vi "sub_result-log.vi"(7 "data":enum16{"header", "result"}(ring), 11 "text":string) -> ()   [LabVIEW 2019]
uses:
  _ctrl/rw.ctl
panel:
  out "path":path
  out "error out":errorcluster
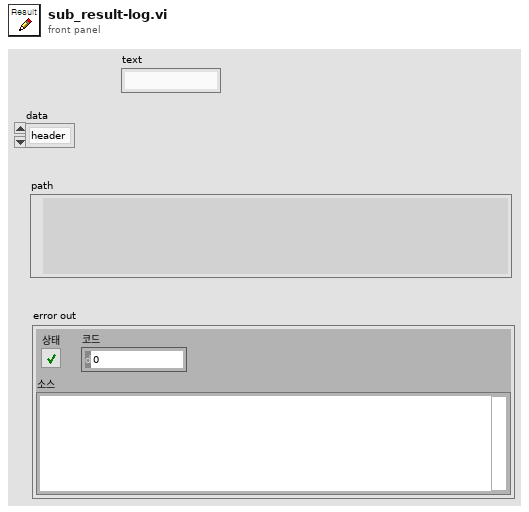
[diagram p1: front panel]
types:
  T1 = typedef "rw.ctl" = enum16{"read", "write"}
  T2 = enum16{"open", "replace", "create", "open or create", "replace or create", "replace or create with confirmation"}
  T3 = typedef "config_aging.ctl" = cluster{"Setting":T4, "TestName":string, "Result path":path, "파일 생성 주기[N]":u8, "Test Specs":T5}
  T4 = typedef "Setting_reg.ctl" = cluster{"제어 전압[V]":dbl, "출력전압[V]":dbl, "전류[A]":dbl, "출력전류[A]":dbl, "ON[초]":dbl, "OFF[초]":dbl, "Irms 허용치 from ":dbl, "Irms 허용치 to":dbl, "AO Delay ms":u32, "Log":path, "result":path}
  T5 = typedef "Breakdown-Spec.ctl" = cluster{"제어단 단선 Irms[mA](이하)":dbl, "제어단 특성 전류 Irms[mA] Max":dbl, "제어단 특성 전류 Irms[mA] Min":dbl, "출력단 단선 Irms[mA](이하)":dbl, "출력단 특성 전류 Irms[mA]  Max":dbl, "출력단 특성전류 Irms[mA]  Min":dbl, "온도[degree]":dbl}
  T6 = typedef "Testing-info.ctl" = cluster{"전체채널수":u8, "현재채널번호":u8, "Irms":dbl, "입력전압":dbl, "입력전류":dbl, "출력전압":dbl, "출력전류":dbl, "온도":dbl, "제어단 단선":bool, "제어단 단락":bool, "제어단 특성변화":bool, "출력단 단선":bool, "출력단 단락":bool, "출력단 특성변화":bool, "출력단 전압":bool, "카운트 일치":bool, "Irms 판정":bool, "온도":bool, "테스트 회수":u32, "TestType":T7, "현재회수":u32, "Ch selection":cluster{"1ch":bool, "2ch":bool, "3ch":bool, "4ch":bool, "5ch":bool, "6ch":bool}, "반복":u32, "Path":path, "파일생성주기":u32, "start time":dbl, "stop time":dbl, "현재반복회수":u32, "NG":cluster{"입출력 카운트":bool, "출력전류RMS":bool}}
  T7 = typedef "sequence_single.ctl" = enum16{"Register", "RC", "B1", "B2", "B3"}
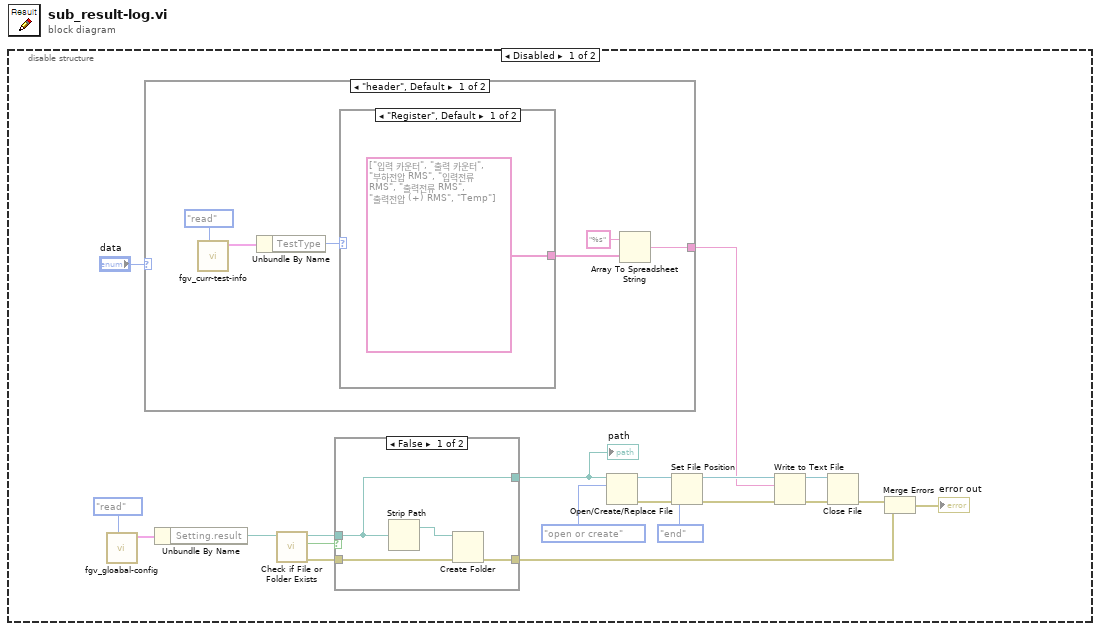
[diagram p0: block diagram]
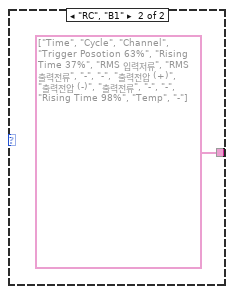
[diagram p2: hidden frame]
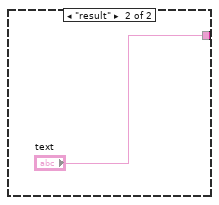
[diagram p3: hidden frame]
diagram:
  n1 = disable-structure shown="Disabled" {
    frame Disabled {
      n2 = call "fgv_gloabal-config.vi"("cmd"=rw."read") -> ("config_aging 2"=w4:T3)  [unwired: 10 in]
      n3 = case shown="\"header\", Default" "data" {
        tunnel: [w25 "text"] -> w2
        frame "header", Default {
          n4 = call "fgv_curr-test-info.vi"("cmd"=rw."read") -> ("현재테스트 정보 2"=w22:T6)  [unwired: 10 in]
          n5 = Unbundle By Name(w22) -> ("TestType"=w21:T7)
          n6 = case shown="\"Register\", Default" w21 {
            tunnel: [string[] ["입력 카운터", "출력 카운터", "부하전압 RMS", "입력전류 RMS", "출력전류 RMS", "출력전압 (+) RMS", "Temp"] string[] ["Time", "Cycle", "Channel", "Trigger Posotion 63%", "Rising Time 37%", "RMS 입력저류", "RMS 출력전류", "-", "-", "출력전압 (+)", "출력전압 (-)", "출력전류", "-", "-", "Rising Time 98%", "Temp", "-"]] -> w26
            frame "Register", Default {
            }
            frame "RC", "B1" {
            }
          }
          n7 = Array To Spreadsheet String(array=w26, 3:"%s" ("format string")) -> (spreadsheet string=w25:string)  [unwired: 1 in]
        }
        frame "result" {
        }
      }
      n8 = Unbundle By Name(w4) -> ("Setting.result"=w3:path)
      n9 = call <vilib>:"Check if File or Folder Exists.vi"("path"=w3) -> ("error out"=w10:errorcluster, "file or folder exists?"=w11:bool, "dup path"=w20:path)  [unwired: 8 in]
      n10 = case shown="False" w11 {
        tunnel: w20 -> [w31 w35]
        tunnel: [w31 w35] -> w6
        tunnel: w10 -> [w33 w34]
        tunnel: [w32 w34] -> w8
        frame False {
          n11 = Strip Path(path=w31) -> (stripped path=w30:path)  [unwired: 1 out]
          n12 = Create Folder(path (use dialog)=w30, error in=w33) -> (error out=w32:errorcluster)  [unwired: 1 in, 2 out]
        }
        frame True {
        }
      }
      "path" <- w6
      n13 = Open/Create/Replace File(file path (use dialog)=w6, operation (0:open)=T2."open or create" ("동작(0:open)")) -> (refnum out=w18:refnum<file>, error out=w17:errorcluster)  [unwired: 4 in, 1 out]
      n14 = Set File Position(refnum=w18, from (0:start)=enum16{"start", "end", "current"}."end" ("위치(0:start)"), error in=w17) -> (refnum out=w14:refnum<file>, error out=w15:errorcluster)  [unwired: 1 in]
      n15 = Write to Text File(file (use dialog)=w14, text=w2, error in=w15) -> (refnum out=w12:refnum<file>, error out=w13:errorcluster)  [unwired: 1 in, 1 out]
      n16 = Close File(refnum=w12, error in=w13) -> (error out=w9:errorcluster)  [unwired: 1 out]
      n17 = Merge Errors(w9, w8) -> (→"error out":errorcluster)
    }
    frame Enabled {
    }
  }
